vi "Load PTU File Information.vi"(8 "error in (no error)":errorcluster, 11 "File Path":path) -> (0 "error out":errorcluster, 1 "Version":string, 2 "PicoQuant Data File Information":T1, 3 "path (dup)":path, 4 "Data offset (in bytes)":i64, 5 "Magic":string, 6 "size (in bytes)":i64, 7 "elapsed (relative) seconds":dbl)   [LabVIEW 2021, in "PicoQuant.lvlib"]
uses:
  PicoQuant.lvlib
  PicoQuant Data File Information.ctl
  PicoQuant File Information.ctl
  PicoQuant Software Information.ctl
  PicoQuant Remote Request Information.ctl
  PicoQuant Hardware Information.ctl
  PicoQuant Input Channels.ctl
  PicoQuant Markers.ctl
  PicoQuant Modules.ctl
  PicoQuant Router Channels.ctl
  PicoQuant Measurement Information.ctl
  PicoQuant Image Information.ctl
  PicoQuant Results Format.ctl
  PicoQuant Measurement Results.ctl
  PTU Files.lvlib
  Time/Time.lvlib
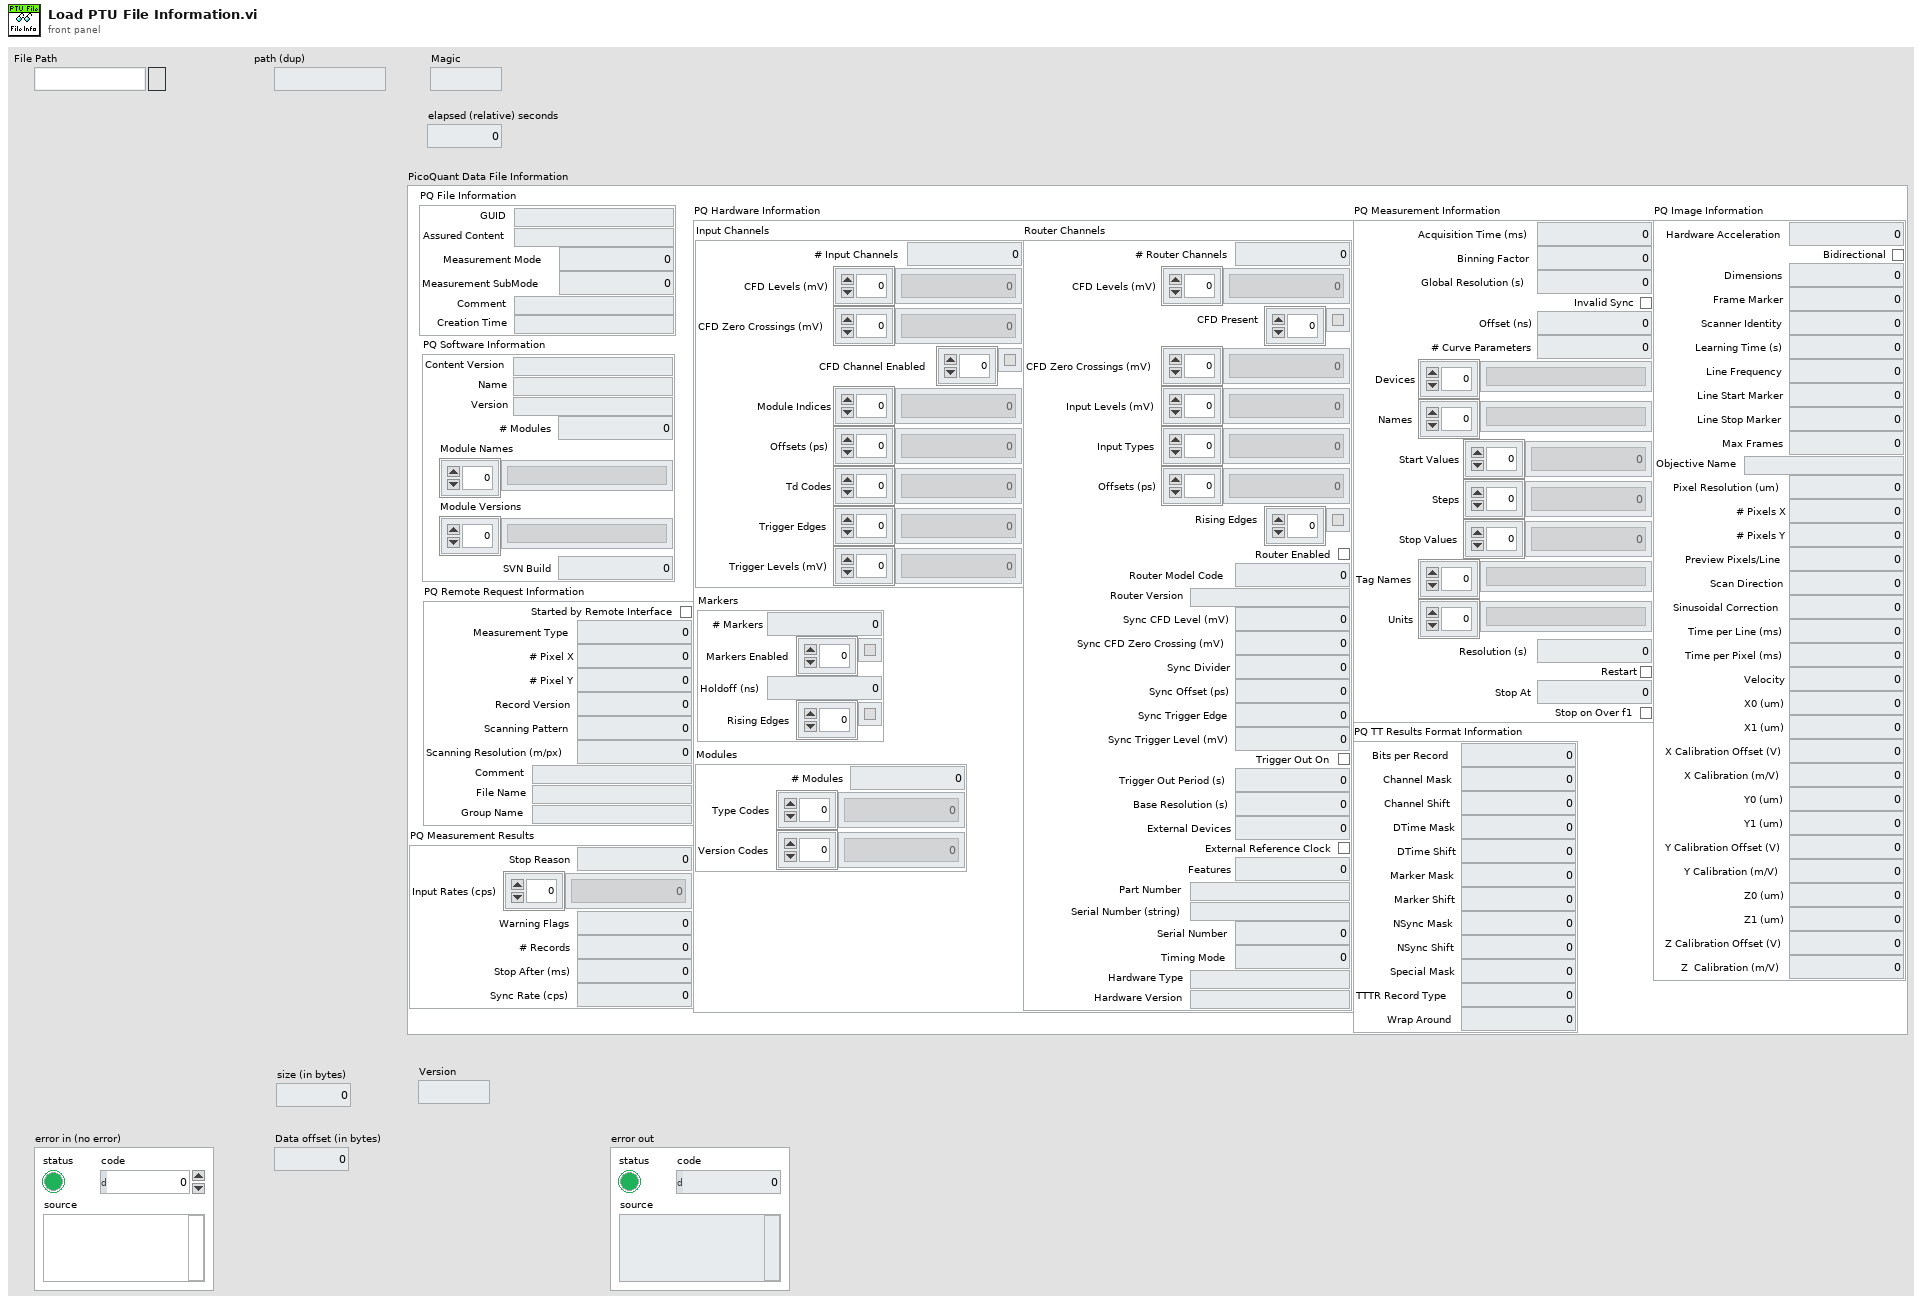
[diagram p1: front panel]
types:
  T1 = typedef "PTU Files.lvlib/PicoQuant Data File Information.ctl" = cluster{"PQ File Information":T2, "PQ Software Information":T3, "PQ Remote Request Information":T4, "PQ Hardware Information":T5, "PQ Measurement Information":T10, "PQ Image Information":T11, "PQ TT Results Format Information":T12, "PQ Measurement Results":T13}
  T2 = typedef "PTU Files.lvlib/PicoQuant File Information.ctl" = cluster{"GUID":string, "Assured Content":string, "Measurement Mode":i64, "Measurement SubMode":i64, "Comment":string, "Creation Time":string}
  T3 = typedef "PTU Files.lvlib/PicoQuant Software Information.ctl" = cluster{"Content Version":string, "Name":string, "Version":string, "# Modules":i64, "Module Names":string[], "Module Versions":string[], "SVN Build":i64}
  T4 = typedef "PTU Files.lvlib/PicoQuant Remote Request Information.ctl" = cluster{"Started by Remote Interface":bool, "Measurement Type":i64, "# Pixel X":i64, "# Pixel Y":i64, "Record Version":i64, "Scanning Pattern":i64, "Scanning Resolution (m/px)":dbl, "Comment":string, "File Name":string, "Group Name":string}
  T5 = typedef "PTU Files.lvlib/PicoQuant Hardware Information.ctl" = cluster{"Input Channels":T6, "Markers":T7, "Modules":T8, "Router Channels":T9}
  T6 = typedef "PTU Files.lvlib/PicoQuant Input Channels.ctl" = cluster{"# Input Channels":i64, "CFD Levels (mV)":i64[], "CFD Zero Crossings (mV)":i64[], "CFD Channel Enabled":bool[], "Module Indices":i64[], "Offsets (ps)":i64[], "Td Codes":i64[], "Trigger Edges":i64[], "Trigger Levels (mV)":i64[]}
  T7 = typedef "PTU Files.lvlib/PicoQuant Markers.ctl" = cluster{"# Markers":i64, "Markers Enabled":bool[], "Holdoff (ns)":i64, "Rising Edges":bool[]}
  T8 = typedef "PTU Files.lvlib/PicoQuant Modules.ctl" = cluster{"# Modules":i64, "Type Codes":i64[], "Version Codes":i64[]}
  T9 = typedef "PTU Files.lvlib/PicoQuant Router Channels.ctl" = cluster{"# Router Channels":i64, "CFD Levels (mV)":i64[], "CFD Present":bool[], "CFD Zero Crossings (mV)":i64[], "Input Levels (mV)":i64[], "Input Types":i64[], "Offsets (ps)":i64[], "Rising Edges":bool[], "Router Enabled":bool, "Router Model Code":i64, "Router Version":string, "Sync CFD Level (mV)":i64, "Sync CFD Zero Crossing (mV)":i64, "Sync Divider":i64, "Sync Offset (ps)":i64, "Sync Trigger Edge":i64, "Sync Trigger Level (mV)":i64, "Trigger Out On":bool, "Trigger Out Period (s)":dbl, "Base Resolution (s)":dbl, "External Devices":i64, "External Reference Clock":bool, "Features":u64, "Part Number":string, "Serial Number (string)":string, "Serial Number":i64, "Timing Mode":i64, "Hardware Type":string, "Hardware Version":string}
  T10 = typedef "PTU Files.lvlib/PicoQuant Measurement Information.ctl" = cluster{"Acquisition Time (ms)":i64, "Binning Factor":i64, "Global Resolution (s)":dbl, "Invalid Sync":bool, "Offset (ns)":u64, "# Curve Parameters":u64, "Devices":string[], "Names":string[], "Start Values":dbl[], "Steps":dbl[], "Stop Values":dbl[], "Tag Names":string[], "Units":string[], "Resolution (s)":dbl, "Restart":bool, "Stop At":u64, "Stop on Over f1":bool}
  T11 = typedef "PTU Files.lvlib/PicoQuant Image Information.ctl" = cluster{"Hardware Acceleration":i64, "Bidirectional":bool, "Dimensions":i64, "Frame Marker":i64, "Scanner Identity":i64, "Learning Time (s)":i64, "Line Frequency":dbl, "Line Start Marker":i64, "Line Stop Marker":i64, "Max Frames":i64, "Objective Name":string, "Pixel Resolution (um)":dbl, "# Pixels X":i64, "# Pixels Y":i64, "Preview Pixels/Line":i64, "Scan Direction":i64, "Sinusoidal Correction":i64, "Time per Line (ms)":dbl, "Time per Pixel (ms)":i64, "Velocity":i64, "X0 (um)":dbl, "X1 (um)":dbl, "X Calibration Offset (V)":dbl, "X Calibration (m/V)":dbl, "Y0 (um)":dbl, "Y1 (um)":dbl, "Y Calibration Offset (V)":dbl, "Y Calibration (m/V)":dbl, "Z0 (um)":dbl, "Z1 (um)":dbl, "Z Calibration Offset (V)":dbl, "Z  Calibration (m/V)":dbl}
  T12 = typedef "PTU Files.lvlib/PicoQuant Results Format.ctl" = cluster{"Bits per Record":i64, "Channel Mask":i64, "Channel Shift ":i64, "DTime Mask":i64, "DTime Shift":i64, "Marker Mask":i64, "Marker Shift":i64, "NSync Mask":i64, "NSync Shift":i64, "Special Mask":i64, "TTTR Record Type":i64, "Wrap Around":i64}
  T13 = typedef "PTU Files.lvlib/PicoQuant Measurement Results.ctl" = cluster{"Stop Reason":i64, "Input Rates (cps)":i64[], "Warning Flags":u64, "# Records":i64, "Stop After (ms)":i64, "Sync Rate (cps)":i64}
  T14 = typedef "PTU Files.lvlib/PicoQuant Header Tag.ctl" = cluster{"TagIdent":string, "TagIndex":i32, "TagType":i32, "TagValue":i64, "TagAuxData":string}
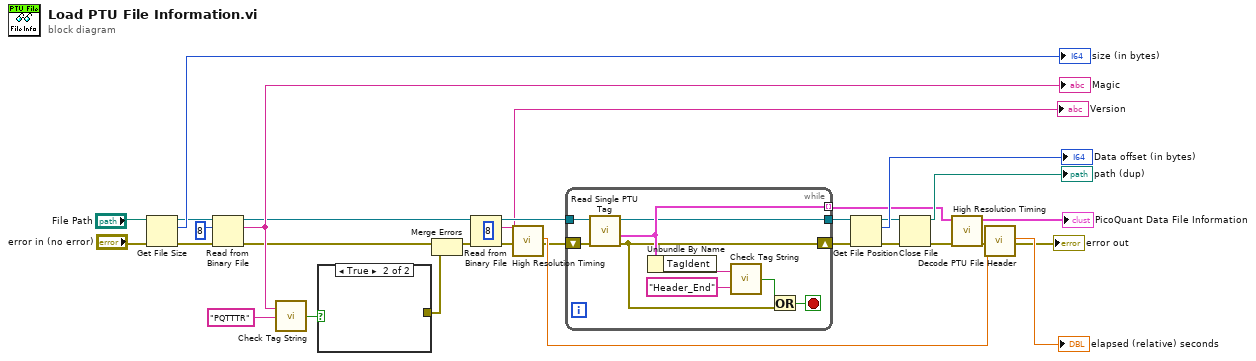
[diagram p0: block diagram]
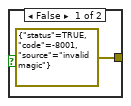
[diagram p2: hidden frame]
diagram:
  n1 = Get File Size(file="File Path", error in="error in (no error)") -> (refnum out=w18:refnum<file>, size (in bytes)=→"size (in bytes)":i64, 0:w19:errorcluster)
  n2 = Read from Binary File(8:w19, 10:8, 11:w18) -> (0:w5:errorcluster, 2:w9:string, 3:w1:refnum<file>)  [unwired: 3 in, 1 out]
  "Magic" <- w9
  n3 = call "Check Tag String.vi"("String 2"="PQTTTR", "String 1"=w9) -> ("equal"=w8:bool)
  n4 = case shown="True" w8 {
    tunnel: [errorcluster {"status"=TRUE, "code"=-8001, "source"="invalid magic"} ("file error status 2") _] -> w7
    frame False {
    }
    frame True {
    }
  }
  n5 = Merge Errors(w5, w7) -> (w6:errorcluster)
  n6 = Read from Binary File(8:w6, 10:8, 11:w1) -> (0:w12:errorcluster, 2:→"Version":string, 3:w10:refnum<file>)  [unwired: 3 in, 1 out]
  n7 = call "High Resolution Timing.vi"("Error In"=w12) -> ("elapsed (relative) seconds"=w30:dbl, "Error Out"=w15:errorcluster)  [unwired: 16 in, 1 out]
  n8 = while {
    shift-left: w15 -> [w40]
    shift-right: [w33] -> w14
    tunnel: w10 -> [w37]
    tunnel: [w35] -> w13 mode=indexing
    tunnel: [w34] -> w22
    stop <- w41 stop-if-true
    n9 = call "Read Single PTU Tag.vi"("error in"=w40, "refnum"=w37) -> ("error out"=w33:errorcluster, "PicoQuant Tag"=w35:T14, "refnum out"=w34:refnum<file>)  [unwired: 7 in]
    n10 = Unbundle By Name(w35) -> ("TagIdent"=w36:string)
    n11 = call "Check Tag String.vi"("String 2"="Header_End", "String 1"=w36) -> ("equal"=w38:bool)
    n12 = Or(x=w38, y=w33) -> (x .or. y?=w41:bool)
  }
  n13 = Get File Position(4:w14, 7:w22) -> (0:w21:errorcluster, 2:→"Data offset (in bytes)":i64, 3:w23:refnum<file>)
  n14 = Close File(refnum=w23, error in=w21) -> (path=→"path (dup)":path, error out=w20:errorcluster)
  n15 = call "Decode PTU File Header.vi"("error in (no error)"=w20, "Tag Array"=w13) -> ("error out"=w28:errorcluster, "PicoQuant Data File Information"=→"PicoQuant Data File Information":T1)  [unwired: 7 in, 1 out]
  n16 = call "High Resolution Timing.vi"("relative seconds (NaN)"=w30, "Error In"=w28) -> ("elapsed (relative) seconds"=→"elapsed (relative) seconds":dbl, "Error Out"=→"error out":errorcluster)  [unwired: 15 in, 1 out]
